vi "Read Q.vi"(8 "error in (no error)":errorcluster, 11 "RFID system in":refnum<class "RFID system.lvclass">) -> (0 "error out":errorcluster, 2 "Q":dbl, 3 "RFID system out":refnum<class "RFID system.lvclass">)   [LabVIEW 2019, in "RFID system.lvclass"]
uses:
  RFID system.lvclass
  RFID system.lvclass/RFID system.ctl
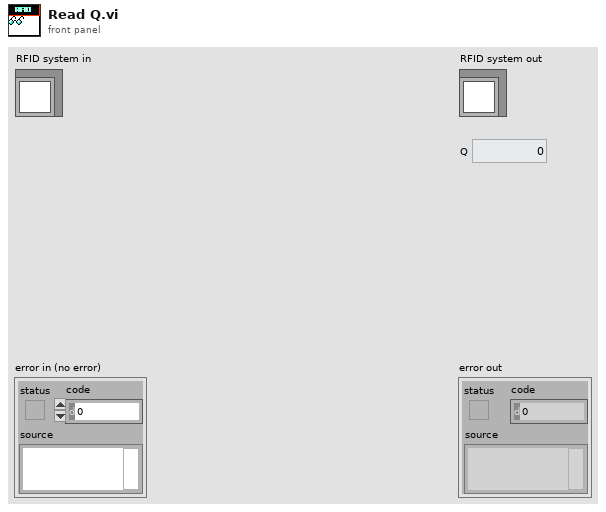
[diagram p1: front panel]
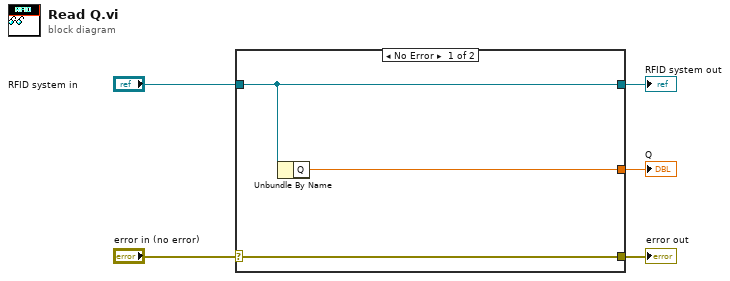
[diagram p0: block diagram]
diagram:
  n1 = case shown="No Error" "error in (no error)" {
    selector: "error in (no error)" -> [w8 w9]
    tunnel: [w8 w9] -> w4
    tunnel: [w7 w10] -> w2
    tunnel: "RFID system in" -> [w7 w10]
    tunnel: [w6 _] -> w1
    frame No Error {
      n2 = Unbundle By Name(w7) -> ("Q"=w6:dbl)
    }
    frame Error {
    }
  }
  "error out" <- w4
  "RFID system out" <- w2
  "Q" <- w1
